vi "AlliGator Update Phasor Harmonic Orders.vi"(8 "Error In":errorcluster, 11 "Stored Phasor Harmonics in":T1[](array[typedef])) -> (0 "Error Out":errorcluster, 3 "Stored Phasor Harmonics out":T1[](array[typedef]))   [LabVIEW 2021]
uses:
  Phasor/Phasor Harmonic Data.ctl
  <userlib>/_OpenG.lib/array/array.llb/Remove Duplicates from 1D Array (Path)__ogtk.vi
  <userlib>/_OpenG.lib/array/array.llb/openg_array.lvlib
  Phasor/Phasor.lvlib
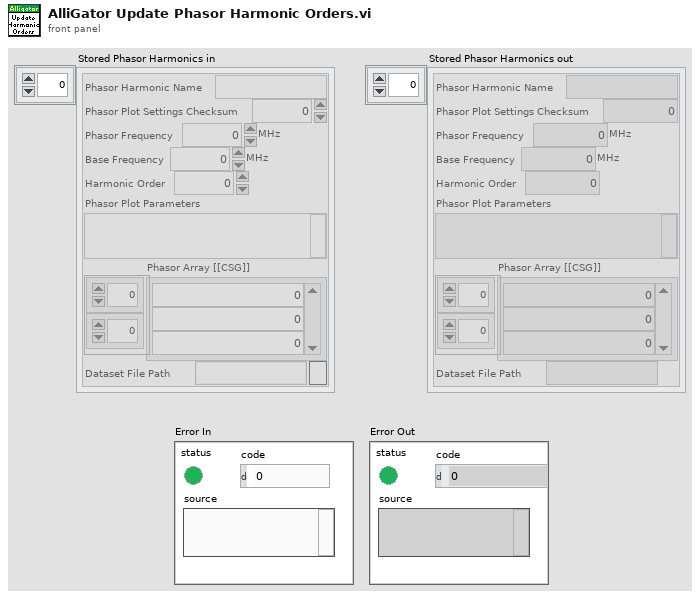
[diagram p1: front panel]
types:
  T1 = typedef "Phasor.lvlib/Phasor Harmonic Data.ctl" = cluster{"Phasor Harmonic Name":string, "Phasor Plot Settings Checksum":u64, "Phasor Frequency":dbl[unit], "Base Frequency":dbl[unit], "Harmonic Order":u8, "Phasor Plot Parameters":string, "Phasor Array [[CSG]]":csg[][], "Dataset File Path":path}
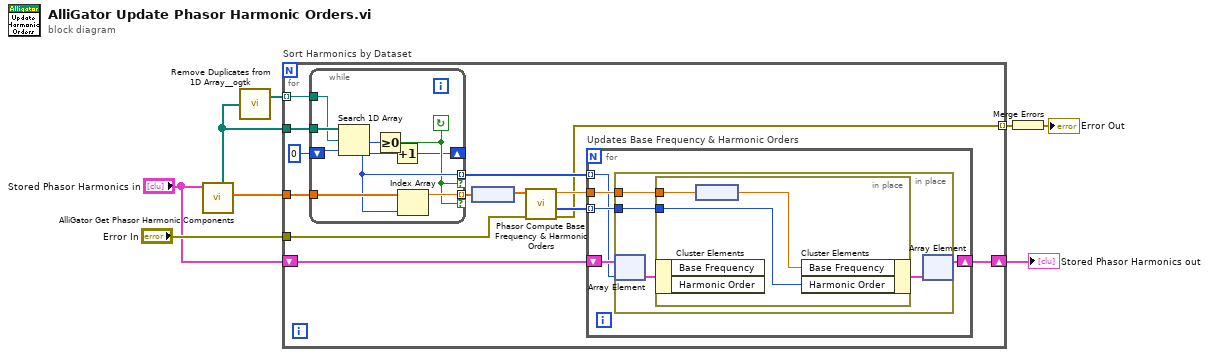
[diagram p0: block diagram]
diagram:
  n1 = call "AlliGator Get Phasor Harmonic Components.vi"("Stored Phasor Harmonics"="Stored Phasor Harmonics in") -> ("Phasor Harmonic Frequencies"=w6:dbl[unit][], "Phasor Harmonic Dataset File Paths"=w7:path[])  [unwired: 4 in, 5 out]
  n2 = call-poly <userlib>:"Remove Duplicates from 1D Array__ogtk.vi"("Input Array"=w7) -> ("Output Array"=w8:path[])  [unwired: 1 out]
  n3 = for "Sort Harmonics by Dataset" {
    tunnel: w8 -> [w20] mode=indexing
    tunnel: w7 -> [w21]
    tunnel: w6 -> [w19]
    tunnel: "Error In" -> [w16]
    shift-right: [w12] -> w3
    shift-left: "Stored Phasor Harmonics in" -> [w13]
    tunnel: [w10] -> w2 mode=indexing
    n4 = while {
      tunnel: w21 -> [w29]
      tunnel: w20 -> [w28]
      tunnel: w19 -> [w27]
      tunnel: [w26] -> w18 mode=indexing if=w23
      tunnel: [w24] -> w11 mode=indexing if=w23
      shift-right: [w22] -> _
      shift-left: 0 ("index of element") -> [w25]
      stop <- w23 continue-if-true
      n5 = Search 1D Array(1D array=w29, element=w28, start index (0)=w25) -> (index of element=w24:i32)
      n6 = Greater Or Equal To 0?(x=w24) -> (x >= 0?=w23:bool)
      n7 = Increment(x=w24) -> (x+1=w22:i32)
      n8 = Index Array(array=w27, index=w24) -> (element=w26:dbl[unit])
    }
    n9 = node(w18) -> (w17:dbl[])
    n10 = call "Phasor Compute Base Frequency & Harmonic Orders.vi"("Error In"=w16, "Frequency Array"=w17) -> ("Error Out"=w10:errorcluster, "Harmonic Orders"=w14:i32[], "Base Frequency"=w15:dbl)  [unwired: 7 in]
    n11 = for "Updates Base Frequency & Harmonic Orders" {
      tunnel: w15 -> [w32]
      tunnel: w14 -> [w31] mode=indexing
      shift-right: [w33] -> w12
      shift-left: w13 -> [w34]
      tunnel: w11 -> [w30] mode=indexing
      n12 = in-place {
        in-place-border: w32 -> [w37]
        in-place-border: w31 -> [w36]
        n13 = in-place-array #1(w34, w30) -> (w38:T1)
        n14 = in-place {
          in-place-border: w37 -> [w41]
          in-place-border: w36 -> [w39]
          n15 = in-place-cluster #2(w38) -> ()  [unwired: 2 out]
          n16 = node(w41) -> (w40:dbl[unit])
          n17 = in-place-cluster #2("Base Frequency"=w40, "Harmonic Order"=w39) -> (w35:T1)
        }
        n18 = in-place-array #1(w35) -> (w33:T1[])  [unwired: 1 out]
      }
    }
  }
  "Stored Phasor Harmonics out" <- w3
  n19 = Merge Errors(w2) -> (→"Error Out":errorcluster)
